vi "DefocussedImage.vi"(0 "Path in":refnum<vi>, 1 "reference":refnum<vi>, 2 "Boolean":bool, 7 "reference 2":refnum<vi>, 9 "reference 3":refnum<vi>, 11 "error in (no error)":errorcluster, 12 "reference 4":refnum<vi>, 13 "reference 5":refnum<vi>) -> (4 "camout":i32[](array[numeric]), 15 "error out":errorcluster)   [LabVIEW 2009]
uses:
  lib/System Files/user.lib/atmcd32d.llb/Error Code Enum typedef.ctl
  ccdChipPixels.vi
  GlobalSetGetConfigureCamera.vi
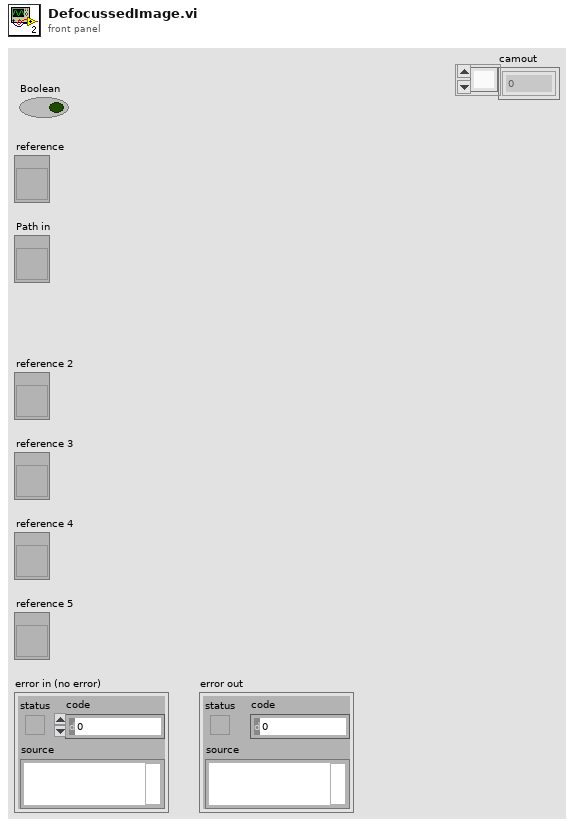
[diagram p1: front panel]
types:
  T1 = cluster{"X-Position":dbl, "Y-Position":dbl, "Z-Position":dbl}
  T2 = typedef "Error Code Enum typedef.ctl" = enum32{"N/A (0)", "DRV_ERROR_CODES", "DRV_SUCCESS", "DRV_VXDNOTINSTALLED", "DRV_ERROR_SCAN", "DRV_ERROR_CHECK_SUM", "DRV_ERROR_FILELOAD", "DRV_UNKNOWN_FUNC", "DRV_ERROR_VXD_INIT", "DRV_ERROR_ADDRESS", "DRV_ERROR_PAGELOCK", "DRV_ERROR_PAGEUNLOCK", "DRV_ERROR_BOARDTEST", "DRV_ERROR_ACK", "DRV_ERROR_UP_FIFO", "DRV_ERROR_PATTERN", "N/A (16)", "DRV_ACQUISITION_ERRORS", "DRV_ACQ_BUFFER", "DRV_ACQ_DOWNFIFO_FULL", "DRV_PROC_UNKONWN_INSTRUCTION", "DRV_ILLEGAL_OP_CODE", "DRV_KINETIC_TIME_NOT_MET", "DRV_ACCUM_TIME_NOT_MET", "DRV_NO_NEW_DATA", "N/A (25)", "DRV_SPOOLERROR", "N/A (27)", "N/A (28)", "N/A (29)", "N/A (30)", "N/A (31)", "N/A (32)", "DRV_TEMPERATURE_CODES", "DRV_TEMPERATURE_OFF", "DRV_TEMPERATURE_NOT_STABILIZED", "DRV_TEMPERATURE_STABILIZED", "DRV_TEMPERATURE_NOT_REACHED", "DRV_TEMPERATURE_OUT_RANGE", "DRV_TEMPERATURE_NOT_SUPPORTED", "DRV_TEMPERATURE_DRIFT", "N/A (41)", "N/A (42)", "N/A (43)", "N/A (44)", "N/A (45)", "N/A (46)", "N/A (47)", "N/A (48)", "DRV_GENERAL_ERRORS", "DRV_INVALID_AUX", "DRV_COF_NOTLOADED", "DRV_FPGAPROG", "DRV_FLEXERROR", "DRV_GPIBERROR", "N/A (55)", "N/A (56)", "N/A (57)", "N/A (58)", "N/A (59)", "N/A (60)", "N/A (61)", "N/A (62)", "N/A (63)", "DRV_DATATYPE", "DRV_DRIVER_ERRORS", "DRV_P1INVALID", "DRV_P2INVALID", "DRV_P3INVALID", "DRV_P4INVALID", "DRV_INIERROR", "DRV_COFERROR", "DRV_ACQUIRING", "DRV_IDLE", "DRV_TEMPCYCLE", "DRV_NOT_INITIALIZED", "DRV_P5INVALID", "DRV_P6INVALID", "DRV_INVALID_MODE", "DRV_INVALID_FILTER", "DRV_I2CERRORS", "DRV_I2CDEVNOTFOUND", "DRV_I2CTIMEOUT", "DRV_P7INVALID", "N/A (84)", "N/A (85)", "N/A (86)", "N/A (87)", "N/A (88)", "N/A (89)", "DRV_IOCERROR", "DRV_VRMVERSIONERROR"}
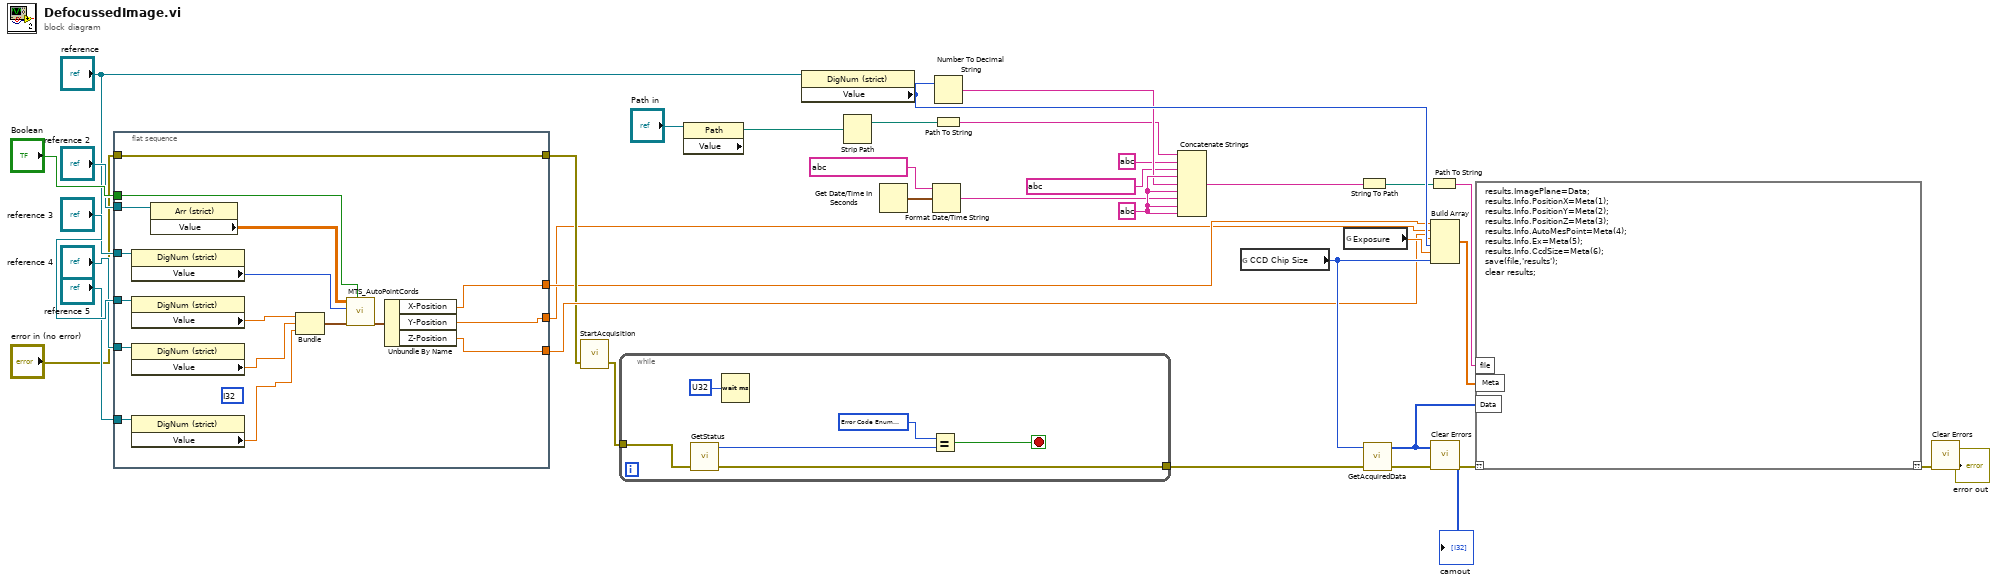
[diagram p0: block diagram]
diagram:
  w21 = string ? ("string")
  n1 = flat-sequence {
    tunnel: "Boolean" -> [w43]
    tunnel: "error in (no error)" -> [w49]
    tunnel: [w49] -> w27
    tunnel: [w38] -> w1
    tunnel: [w39] -> w2
    tunnel: [w37] -> w28
    tunnel: "reference 2" -> [w48]
    tunnel: "reference 3" -> [w47]
    tunnel: "reference 4" -> [w46]
    tunnel: "reference 5" -> [w45]
    tunnel: "reference" -> [w44]
    frame #0 {
      (unwired) i32 ?
      n2 = property class="DigNum (strict)"(reference=w44) -> ("Value"=w53:i32)  [unwired: 1 in, 2 out]
      n3 = property class="DigNum (strict)"(reference=w47) -> ("Value"=w40:dbl)  [unwired: 1 in, 2 out]
      n4 = property class="DigNum (strict)"(reference=w46) -> ("Value"=w41:dbl)  [unwired: 1 in, 2 out]
      n5 = property class="DigNum (strict)"(reference=w45) -> ("Value"=w42:dbl)  [unwired: 1 in, 2 out]
      n6 = property class="Arr (strict)"(reference=w48) -> ("Value"=w52:dbl[][])  [unwired: 1 in, 2 out]
      n7 = Bundle("Value"=w40, "Value"=w41, "Value"=w42) -> (w51:cluster{"Value":dbl, "Value":dbl, "Value":dbl})  [unwired: 1 in]
      n8 = call "MTS_AutoPointCords.vi"("Is Auto Point"=w43, "Cords In"=w51, "Next Auto Measure Point"=w53, "Pattern"=w52) -> ("Cords"=w50:T1)  [unwired: 7 in]
      n9 = Unbundle By Name(w50) -> ("X-Position"=w39:dbl, "Y-Position"=w38:dbl, "Z-Position"=w37:dbl)
    }
  }
  n10 = call "StartAcquisition.vi"("error in (no error)"=w27) -> ("error out"=w10:errorcluster)  [unwired: 1 in, 1 out]
  n11 = while {
    tunnel: w10 -> [w54]
    tunnel: [w57] -> w12
    stop <- w56 stop-if-true
    n12 = call "GetStatus.vi"("error in (no error)"=w54) -> ("error out"=w57:errorcluster, "status"=w58:T2)  [unwired: 2 in, 1 out]
    n13 = Wait (ms)(milliseconds to wait=u32 ?) -> ()  [unwired: 1 out]
    n14 = Equal?(x=T2 ? ("status"), y=w58) -> (x = y?=w56:bool)
  }
  n15 = property on="Property Node" class="Path"(reference="Path in") -> ("Value"=w22:path)  [unwired: 1 in, 2 out]
  n16 = property class="DigNum (strict)"(reference="reference") -> ("Value"=w29:i32)  [unwired: 1 in, 2 out]
  n17 = Strip Path(path=w22) -> (stripped path=w14:path)  [unwired: 1 out]
  n18 = Get Date/Time In Seconds() -> (seconds since 1Jan1904=w18:timestamp)
  n19 = Format Date/Time String(time format string (%c)=string ?, seconds (now)=w18) -> (date/time string=w20:string)  [unwired: 1 in]
  n20 = Path To String(path=w14) -> (string=w13:string)
  n21 = Number To Decimal String(number=w29) -> (decimal integer string=w17:string)  [unwired: 1 in]
  n22 = Concatenate Strings(w13, string ? ("string"), string ? ("string"), w21, w17, w21, w20, w21, w21) -> (w24:string)
  n23 = global read "ccdChipPixels.vi" "CCD Chip Size"() -> (w31:i32)
  n24 = global read "GlobalSetGetConfigureCamera.vi" "Exposure"() -> (w30:sgl)
  n25 = String To Path(string=w24) -> (path=w23:path)
  n26 = call "GetAcquiredData.vi"("error in (no error)"=w12, "size"=w31) -> ("error out"=w11:errorcluster, "array"=w36:i32[])  [unwired: 1 in, 1 out]
  "camout" <- w36
  n27 = Path To String(path=w23) -> (string=w25:string)
  n28 = Build Array(w2, w1, w28, w29, w30, w31) -> (w32:dbl[])
  n29 = call <vilib>:"Clear Errors.vi"("error in (no error)"=w11) -> ("error out"=w33:errorcluster)  [unwired: 6 in]
  n30 = script code="results.ImagePlane=Data;\nresults.Info.PositionX=Meta(1);\nresults.Info.PositionY=Meta(2);\nresults.Info.PositionZ=Meta(3);\nresults.Info.AutoMesPoint=Meta(4);\nresults.Info.Ex=Meta(5);\nresults.Info.CcdSize=Meta(6);\nsave(file,'results');\nclear results;"("??"=w33, "Data"=w36, "Meta"=w32, "file"=w25) -> ("??"=w34:errorcluster)
  n31 = call <vilib>:"Clear Errors.vi"("error in (no error)"=w34) -> ("error out"=→"error out":errorcluster)  [unwired: 6 in]
